vi "TagDB-TestMain.vi"() -> ()   [LabVIEW 2017]
uses:
  a1ae43e1-b2e0-48b2-b5bf-09d8c6337ec0.vi
  5d4c14d8-f2b2-4cd0-9f9f-81160b0f88f4.vi
  69a5f5dc-289e-4520-a43d-4a6e53800127.vi
  b9594d6d-a8e1-4e69-b527-0d31d87043e6.vi
  f6a41f1a-46ba-40d5-b8b9-4f6d9d3cd2d0.vi
  src/TagDB/_Support/Change Detector/TagDB dbChanged.vi
  src/TagDB/_Support/DataAccess/data-Write.vi
  src/TagDB/_Support/DataAccess/TagDB Ref to DVR.vi
  src/TagDB/_Support/DataAccess/_NameCacher.vi
  src/TagDB/_Support/URL/TRIM-BOTH-SPACE.vi
  src/TagDB/_Support/Change Detector/TagDB ChangeFlag.vi
  src/TagDB/_Support/DataAccess/_datatypeChecker.vi
  <vilib>/Utility/Data Type/Get Type Information.vi
  src/TagDB/_Support/Error/_[error50000]Invalid DB REF.vi
  src/TagDB/_Support/Error/_[error50002]Invalid DataType.vi
  src/TagDB/TagDB.lvlib
panel:
  out "changed?":bool[](array[boolean])
  in  "Reject New Tag(F)":bool=TRUE
  out "should be datatype error":errorcluster
  out "should be no tag error":errorcluster
  out "Raw name":string
  in  "Type":cluster{"Numeric":i32, "String":string}
  in  "Stop":bool
  out "Value":cluster{"Numeric":i32, "String":string}
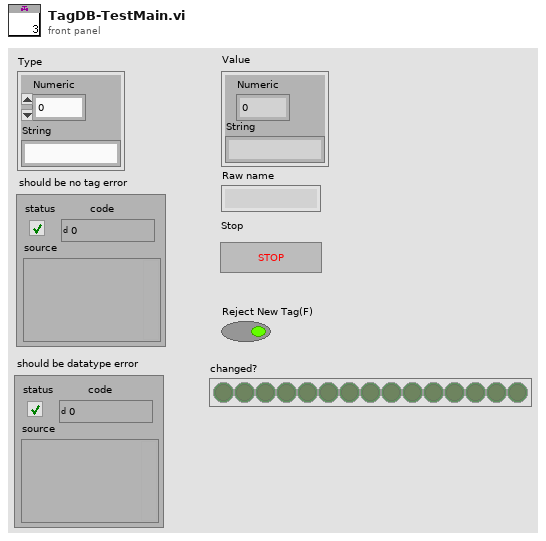
[diagram p1: front panel]
types:
  T1 = typedef "TagDB.lvlib/TagDB.ctl" = refnum<k1>
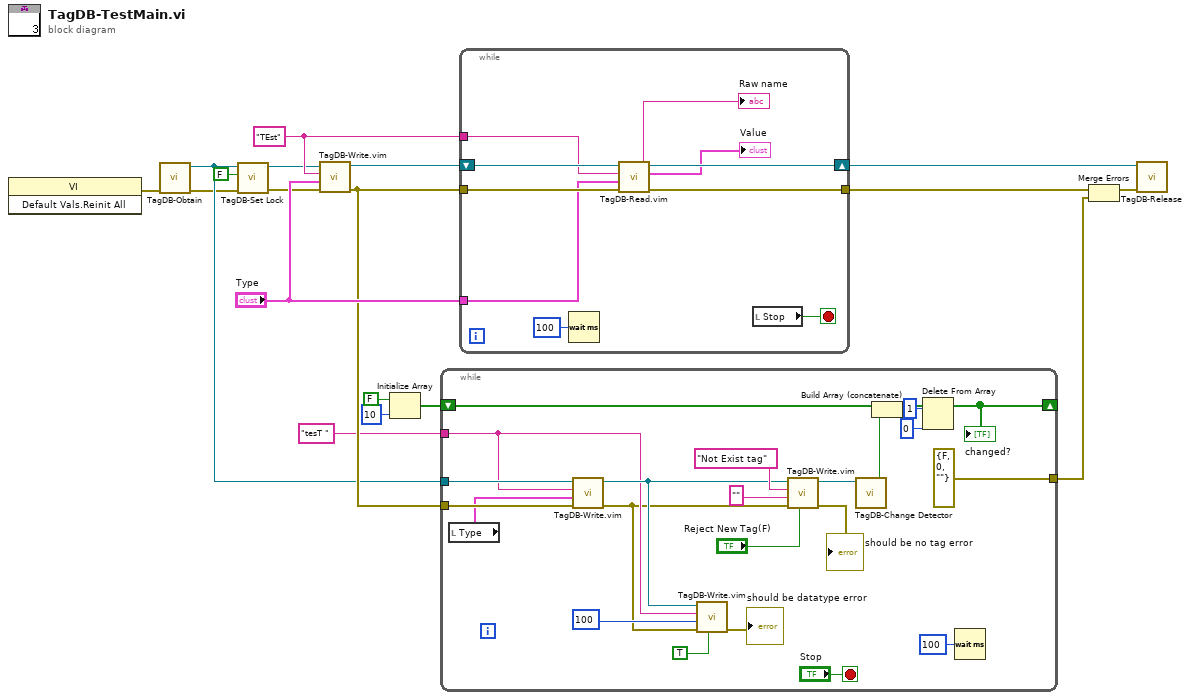
[diagram p0: block diagram]
diagram:
  w14 = "TEst" ("name")
  n1 = invoke class="VI" method="Default Vals.Reinit All"() -> (error out=w10:errorcluster)  [unwired: 3 in, 2 out]
  n2 = call "TagDB-Obtain.vi"("error in (no error)"=w10) -> ("error out"=w4:errorcluster, "TagDB"=w5:T1)  [unwired: 4 in, 1 out]
  n3 = call "TagDB-Set Lock.vi"("error in (no error)"=w4, "Lock?(T)"=FALSE, "TagDB"=w5) -> ("error out"=w3:errorcluster, "TagDB(dup)"=w2:T1)  [unwired: 7 in]
  n4 = call "TagDB-Write.vim"("error in (no error)"=w3, "Value"="Type", "tag"=w14, "TagDB"=w2) -> ("error out"=w13:errorcluster, "TagDB(dup)"=w18:T1)  [unwired: 5 in, 1 out]
  n5 = Initialize Array(FALSE, 10 ("dimension size")) -> (w6:bool[])
  n6 = while {
    tunnel: w5 -> [w39]
    tunnel: "tesT " ("name") -> [w32]
    tunnel: w13 -> [w38]
    tunnel: [errorcluster {"status"=FALSE, "code"=0, "source"=""} ("error out")] -> w11
    shift-right: [w23] -> _
    shift-left: w6 -> [w26]
    stop <- "Stop" stop-if-true
    n7 = local read "Type"() -> (w20:cluster{"Numeric":i32, "String":string})
    n8 = call "TagDB-Write.vim"("error in (no error)"=w38, "Value"=w20, "tag"=w32, "TagDB"=w39) -> ("error out"=w30:errorcluster, "TagDB(dup)"=w33:T1)  [unwired: 5 in, 1 out]
    n9 = call "TagDB-Write.vim"("Reject New Tag(F)"=TRUE, "error in (no error)"=w30, "Value"=u32 100 ("milliseconds to wait"), "tag"=w32, "TagDB"=w33) -> ("error out"=→"should be datatype error":errorcluster)  [unwired: 4 in, 2 out]
    n10 = call "TagDB-Write.vim"("Reject New Tag(F)"="Reject New Tag(F)", "error in (no error)"=w30, "Value"="" ("name"), "tag"="Not Exist tag" ("name"), "TagDB"=w33) -> ("error out"=→"should be no tag error":errorcluster, "TagDB(dup)"=w27:T1)  [unwired: 4 in, 1 out]
    n11 = call-poly "TagDB-Change Detector.vi"("DB Ref"=w27) -> ("changed?"=w25:bool)  [unwired: 8 in, 2 out]
    n12 = Build Array (concatenate)(w26, w25) -> (w24:bool[])
    n13 = Delete From Array(array=w24, length=1, index=0) -> (array with subset deleted=w23:bool[])  [unwired: 1 out]
    "changed?" <- w23
    n14 = Wait (ms)(milliseconds to wait=u32 100) -> ()  [unwired: 1 out]
  }
  n15 = while {
    tunnel: w14 -> [w47]
    tunnel: "Type" -> [w46]
    shift-right: [w49] -> w17
    shift-left: w18 -> [w51]
    tunnel: w13 -> [w50]
    tunnel: [w48] -> w16
    stop <- w44 stop-if-true
    n16 = Wait (ms)(milliseconds to wait=u32 100) -> ()  [unwired: 1 out]
    n17 = call "TagDB-Read.vim"("error in (no error)"=w50, "Type(empty to read as variant)"=w46, "name"=w47, "TagDB"=w51) -> ("error out"=w48:errorcluster, "Value"=→"Value":cluster{"Numeric":i32, "String":string}, "TagDB(dup)"=w49:T1, "Raw name"=→"Raw name":string)  [unwired: 2 in, 2 out]
    n18 = local read "Stop"() -> (w44:bool)
  }
  n19 = Merge Errors(w16, w11) -> (w12:errorcluster)
  n20 = call "TagDB-Release.vi"("error in (no error)"=w12, "TagDB"=w17) -> ()  [unwired: 9 in, 1 out]
